vi "system_checks.vi"(8 "error in (no error)":errorcluster, 11 "Experiment in":refnum<class "Experiment.lvclass">) -> (0 "error out":errorcluster, 3 "Experiment out":refnum<class "Experiment.lvclass">)   [LabVIEW 2013, in "Experiment.lvclass"]
uses:
  Experiment.lvclass
  Experiment.lvclass/Experiment.ctl
  TTL_input/TTL_input.lvclass
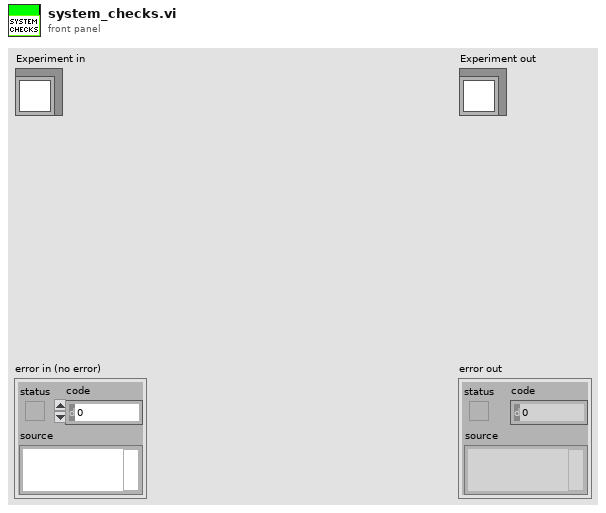
[diagram p1: front panel]
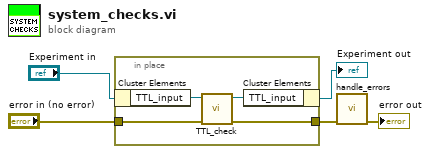
[diagram p0: block diagram]
diagram:
  n1 = in-place {
    in-place-border: "error in (no error)" -> [w7]
    in-place-border: [w6] -> w1
    n2 = in-place-cluster #1("Experiment in") -> ("TTL_input"=w9:refnum<class "TTL_input.lvclass">)
    n3 = call-dynamic "TTL_check.vi"("error in (no error)"=w7, "TTL_input in"=w9) -> ("error out"=w6:errorcluster, "TTL_input out"=w8:refnum<class "TTL_input.lvclass">)  [unwired: 8 in]
    n4 = in-place-cluster #1("TTL_input"=w8) -> (→"Experiment out":refnum<class "Experiment.lvclass">)
  }
  n5 = call "handle_errors.vi"("error in (no error)"=w1) -> ("error out"=→"error out":errorcluster)  [unwired: 10 in]
